vi "WriteSizeNchwMat.vi"   [LabVIEW 2020, in "OpenLvVision_OpenCv.lvlib"]
uses:
  OpenLvVision_OpenCv.lvlib
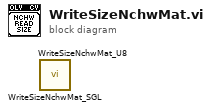
[diagram p0: block diagram]
diagram:
  n1 = call "WriteSizeNchwMat_SGL.vi"() -> ()  [unwired: 10 in, 2 out]
  n2 = call "WriteSizeNchwMat_U8.vi"() -> ()  [unwired: 10 in, 2 out]
